vi "PID_MF.vi"(8 "Time to wait between updates B  (ms)":dbl, 9 "Target Massflow":dbl, 10 "Time to wait between updates A  (ms)":dbl, 11 "Real massflow":dbl) -> (2 "Corrected fan control voltage":dbl, 3 "Corrected servo angle":dbl)   [LabVIEW 2023]
uses:
  <vilib>/addons/control/pid/pid.llb/PID (DBL).vi
  <vilib>/addons/control/pid/NI_PID_pid.lvlib
  <vilib>/addons/control/pid/NI_PID_autopid.lvlib
panel:
  in  "Autotune":bool
  out "Waveform Chart":dbl(graph)
  in  "PID gains A":T1={"proportional gain (Kc)"=1.0, "integral time (Ti, min)"=0.01, "derivative time (Td, min)"=0.0} {"derivative time (Td, min)" format="%.3f"; "integral time (Ti, min)" format="%.3f"; "proportional gain (Kc)" format="%.3f"}
  in  "output range A (degrees)":cluster{"output high":dbl, "output low":dbl}={"output high"=100.0, "output low"=-100.0} {"output low" format="%.2f"; "output high" format="%.2f"}
  in  "output range B (Voltage)":cluster{"output high":dbl, "output low":dbl}={"output high"=100.0, "output low"=-100.0} {"output low" format="%.2f"; "output high" format="%.2f"}
  in  "PID gains B":T1={"proportional gain (Kc)"=1.0, "integral time (Ti, min)"=0.01, "derivative time (Td, min)"=0.0} {"derivative time (Td, min)" format="%.3f"; "integral time (Ti, min)" format="%.3f"; "proportional gain (Kc)" format="%.3f"}
  # "A -> Desired massflow is under 100 m^3/h, control variable is servo"
  # "Not implemented yet"
  # "B -> Desired massflow is above 100 m^3/h, control variable is fan speed"
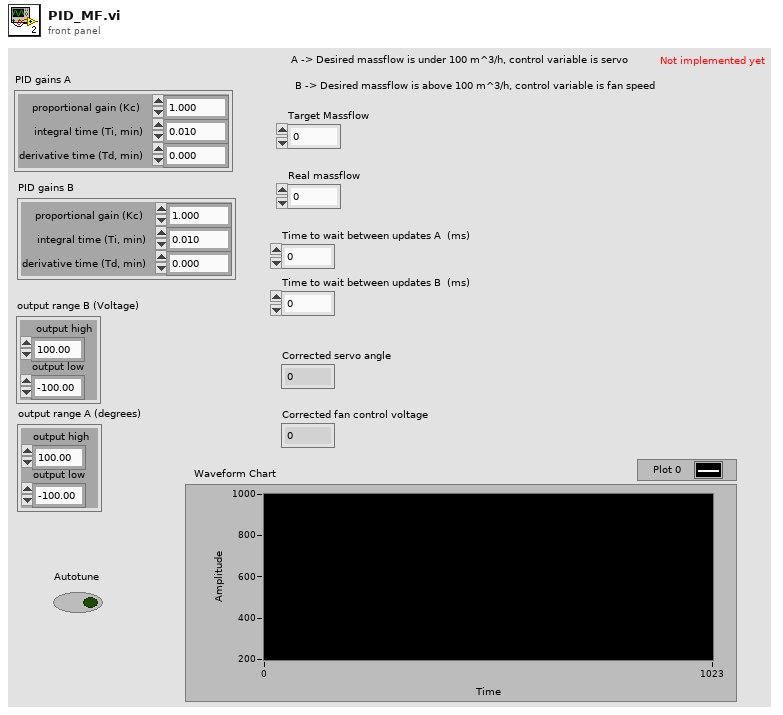
[diagram p1: front panel]
types:
  T1 = cluster{"proportional gain (Kc)":dbl, "integral time (Ti, min)":dbl, "derivative time (Td, min)":dbl}
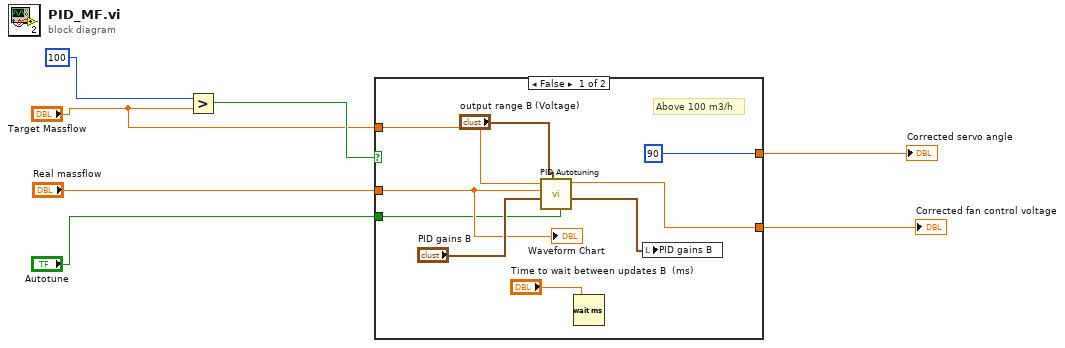
[diagram p0: block diagram]
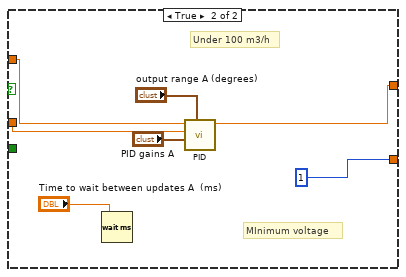
[diagram p2: hidden frame]
diagram:
  n1 = Greater?(x=100, y="Target Massflow") -> (0:w6:bool)
  n2 = case shown="False" w6 {
    tunnel: [w11 1] -> w5
    tunnel: [90 w22] -> w4
    tunnel: "Real massflow" -> [w10 w17]
    tunnel: "Target Massflow" -> [w14 w18]
    tunnel: "Autotune" -> [w8 _]
    frame False {
      # "Above 100 m3/h"
      n3 = call <vilib>:"PID Autotuning.vi"("autotune? (F)"=w8, "output range"="output range B (Voltage)", "PID gains"="PID gains B", "process variable"=w10, "setpoint"=w14) -> ("PID gains out"=w9:T1, "output"=w11:dbl)  [unwired: 3 in, 2 out]
      n4 = Wait (ms)(milliseconds to wait="Time to wait between updates B  (ms)") -> ()  [unwired: 1 out]
      n5 = local write "PID gains B"(w9) -> ()
      "Waveform Chart" <- w10
    }
    frame True {
      # "MInimum voltage"
      # "Under 100 m3/h"
      n6 = Wait (ms)(milliseconds to wait="Time to wait between updates A  (ms)") -> ()  [unwired: 1 out]
      n7 = call-poly <vilib>:"PID.vi"("output range"="output range A (degrees)", "PID gains"="PID gains A", "process variable"=w17, "setpoint"=w18) -> ("output"=w22:dbl)  [unwired: 6 in, 1 out]
    }
  }
  "Corrected servo angle" <- w4
  "Corrected fan control voltage" <- w5
